vi "Do.vi"(8 "error in (no error)":errorcluster, 10 "Actor in":refnum<class "Actor.lvclass">, 11 "DNL_Message Template":refnum<class "StartStop Msg.lvclass">) -> (0 "error out":errorcluster, 2 "Actor out":refnum<class "Actor.lvclass">)   [LabVIEW 2020, in "StartStop Msg.lvclass"]
doc: "This VI delivers the message to the actor by calling the appropriate method(s) on the actor."
uses:
  StartStop Msg.lvclass
  <vilib>/ActorFramework/Actor/Actor.lvclass
  9ef47adc-f318-494c-9b8b-6df3216d6863.vi
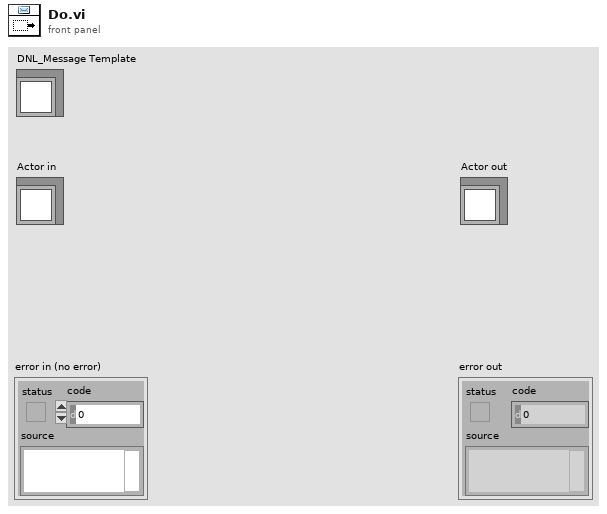
[diagram p1: front panel]
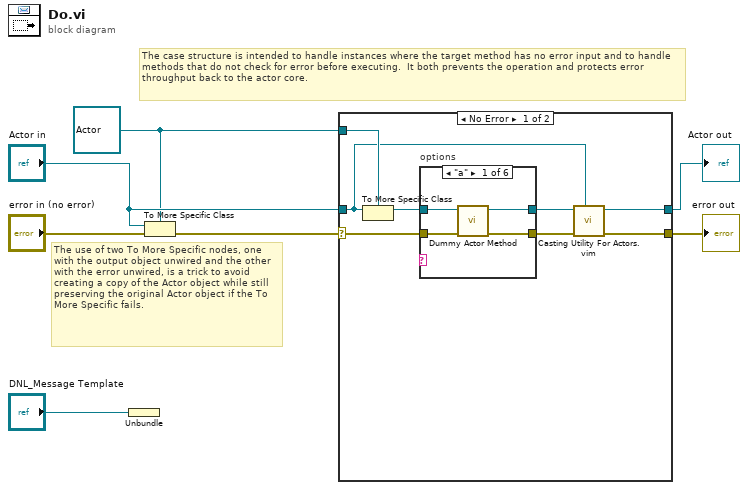
[diagram p0: block diagram]
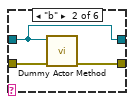
[diagram p2: hidden frame]
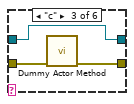
[diagram p3: hidden frame]
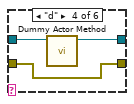
[diagram p4: hidden frame]
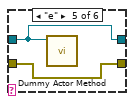
[diagram p5: hidden frame]
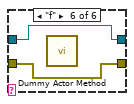
[diagram p6: hidden frame]
diagram:
  w1 = refnum<class "Actor.lvclass"> refnum ("Actor in")
  # "The use of two To More Specific nodes, one with the output object unwired and the other with the error unwired, is a trick to avoid creating a copy of the Actor object while still preserving the original Actor object if the To More Specific fails."
  # "The case structure is intended to handle instances where the target method has no error input and to handle methods that do not check for error before executing.  It both prevents the operation and protects error throughput back to the actor core."
  n1 = Unbundle("DNL_Message Template") -> ()  [unwired: 1 out]
  n2 = To More Specific Class(target class=w1, reference="Actor in", error in="error in (no error)") -> (error out=w5:errorcluster)  [unwired: 1 out]
  n3 = case shown="No Error" w5 {
    selector: w5 -> [w15 w34]
    tunnel: [w9 w34] -> w4
    tunnel: [w10 w33] -> w3
    tunnel: "Actor in" -> [w12 w33]
    tunnel: w1 -> [w13 _]
    frame No Error {
      n4 = To More Specific Class(target class=w13, reference=w12) -> (specific class reference=w14:refnum<class "Actor.lvclass">)  [unwired: 1 in, 1 out]
      n5 = case "options" shown="\"a\"" {
        selector: _ -> [_ _ _ _ _ _]
        tunnel: [w19 w22 w25 w28 w29 w31] -> w8
        tunnel: [w18 w20 w23 w26 w30 w32] -> w11
        tunnel: w15 -> [w17 w21 w24 w28 w29 w31]
        tunnel: w14 -> [w16 w20 w23 w27 w30 w32]
        frame "a" {
          n6 = call <resource>:"Dummy Actor Method.vi"("error in (no error)"=w17, "Actor in"=w16) -> ("error out"=w19:errorcluster, "Actor out"=w18:refnum<class "Actor.lvclass">)  [unwired: 8 in]
        }
        frame "b" {
          n7 = call <resource>:"Dummy Actor Method.vi"("error in (no error)"=w21, "Actor in"=w20) -> ("error out"=w22:errorcluster)  [unwired: 8 in, 1 out]
        }
        frame "c" {
          n8 = call <resource>:"Dummy Actor Method.vi"("error in (no error)"=w24) -> ("error out"=w25:errorcluster)  [unwired: 9 in, 1 out]
        }
        frame "d" {
          n9 = call <resource>:"Dummy Actor Method.vi"("Actor in"=w27) -> ("Actor out"=w26:refnum<class "Actor.lvclass">)  [unwired: 9 in, 1 out]
        }
        frame "e" {
          n10 = call <resource>:"Dummy Actor Method.vi"("Actor in"=w30) -> ()  [unwired: 9 in, 2 out]
        }
        frame "f" {
          n11 = call <resource>:"Dummy Actor Method.vi"() -> ()  [unwired: 10 in, 2 out]
        }
      }
      n12 = call "Casting Utility For Actors.vim"("type"=w12, "error in (no error)"=w8, "Actor in"=w11) -> ("error out"=w9:errorcluster, "Actor out"=w10:refnum<class "Actor.lvclass">)  [unwired: 7 in]
    }
    frame Error {
      # "If type check fails, pass the original object out again."
    }
  }
  "error out" <- w4
  "Actor out" <- w3
